vi "QAM Data to String.vi"(8 "error in (no error)":errorcluster, 10 "symbol map 16 QAM":cdb[](array[numeric]), 11 "QAM Data Out":cluster{dbl[], dbl[]}) -> (0 "error out":errorcluster, 3 "Output String":string)   [LabVIEW 2011]
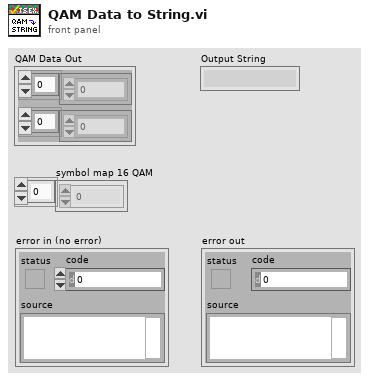
[diagram p1: front panel]
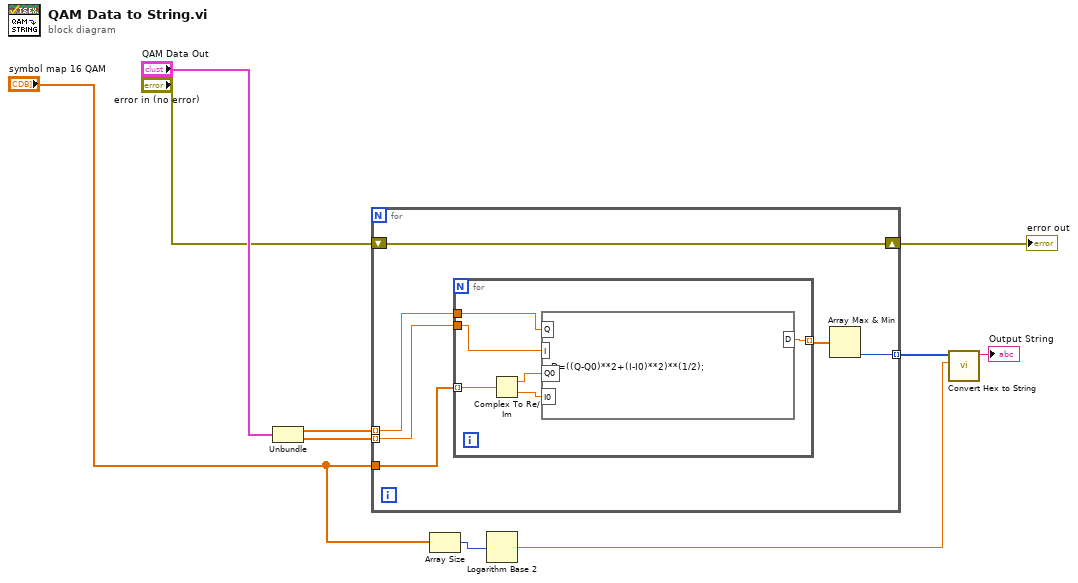
[diagram p0: block diagram]
diagram:
  n1 = Unbundle("QAM Data Out") -> (w4:dbl[], w5:dbl[])
  n2 = for {
    tunnel: w4 -> [w15] mode=indexing
    tunnel: w5 -> [w14] mode=indexing
    tunnel: "symbol map 16 QAM" -> [w16]
    tunnel: [w12] -> w6 mode=indexing
    shift-right: [w11] -> w8
    shift-left: "error in (no error)" -> [w11]
    n3 = for {
      tunnel: w16 -> [w22] mode=indexing
      tunnel: w15 -> [w18]
      tunnel: w14 -> [w19]
      tunnel: [w17] -> w13 mode=indexing
      n4 = Complex To Re/Im(x + iy=w22) -> (x=w21:dbl, y=w20:dbl)
      n5 = formula code="D=((Q-Q0)**2+(I-I0)**2)**(1/2);"("Q"=w18, "I"=w19, "Q0"=w21, "I0"=w20) -> ("D"=w17:dbl)
    }
    n6 = Array Max & Min(array=w13) -> (min index (indices)=w12:i32)  [unwired: 3 out]
  }
  "error out" <- w8
  n7 = Array Size(array="symbol map 16 QAM") -> (size(s)=w2:i32)
  n8 = Logarithm Base 2(1:w2) -> (0:w1:dbl)
  n9 = call "Convert Hex to String.vi"("bits per element"=w1, "Hex Values"=w6) -> ("Output String"=→"Output String":string)  [unwired: 8 in]
